vi "Prober_ProbeTouchdown.vi"(8 "error in (no error)":errorcluster, 11 "SemiProbe in":refnum<class "SemiProbe.lvclass">) -> (0 "error out":errorcluster, 1 "previous Z [µm]":i32, 2 "Z [µm]":i32, 3 "SemiProbe out":refnum<class "SemiProbe.lvclass">)   [LabVIEW 2018, in "SemiProbe.lvclass"]
uses:
  SemiProbe.lvclass
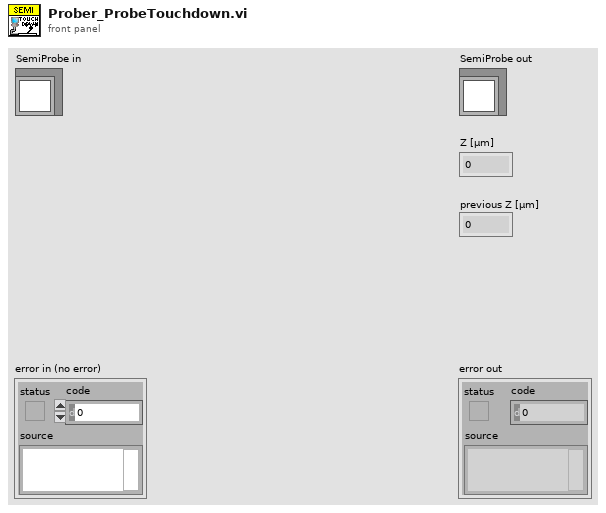
[diagram p1: front panel]
types:
  T1 = enum16{"Move To Load", "Move To Double Separation", "Move To Separation Distance", "Move To Contact", "Execute Contact Search", "Execute Arduino Contact Search"}
  T2 = cluster{"SP Load Less Than Thr?":bool, "SP Load Threshold (um)":dbl, "SP Current Location":cluster{"X (um)":ext, "Y (um)":ext, "Z (um)":ext, "T (degree)":ext}, "SP Chuck Speeds":cluster{"XY Speed (10-100%)":dbl, "Z Speed (10-100%)":dbl, "T Speed (10-100%)":dbl}, "Manual Step Parameters":cluster{"Step in X":bool, "X S-Speed [µm/step]":sgl, "Step in Y":bool, "Y S-Speed [µm/step]":sgl, "Step in Z":bool, "Z S-Speed [µm/step]":sgl, "Step in T":bool, "T S-Speed [mdegree/step]":sgl, "X Increase":bool, "Y Increase?":bool, "Z Increase?":bool, "T Increase?":bool}, "Z Stepper":cluster{"UP/DOWN":bool, "UP/DOWN Speed [µm/step]":i32, "SP Z Step":bool}, "Z Heights Set":bool, "SP Contact Search":cluster{"Contact Circuit":enum16{"12", "1", "2"}, "Speed [1000-10000]":sgl, "Start Height [µm]":sgl, "Search Band [µm]":sgl, "Overdrive [µm]":sgl}, "Separation Distance [µm]":u32, "Contact Height [µm]":u32, "Use Overdrive?":bool, "Touchdown method":enum16{"no feedback", "Arduino edgesense", "SP contact circuit"}, "Arduino Edgesense params":cluster{"touchdown height [µm]":i32, "search band [µm]":u32, "speed [µm/step]":u32, "overdrive [µm]":u32}}
  T3 = enum16{"no feedback", "Arduino edgesense", "SP contact circuit"}
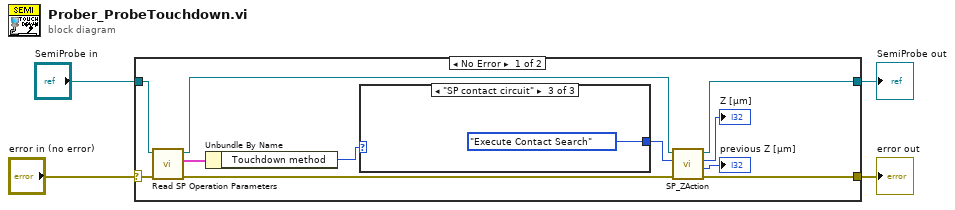
[diagram p0: block diagram]
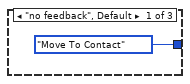
[diagram p2: hidden frame]
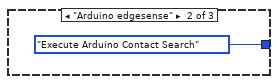
[diagram p3: hidden frame]
diagram:
  n1 = case shown="No Error" "error in (no error)" {
    selector: "error in (no error)" -> [w10 w19]
    tunnel: "SemiProbe in" -> [w9 w20]
    tunnel: [w12 w19] -> w2
    tunnel: [w11 w20] -> w1
    frame No Error {
      n2 = call-dynamic "Read SP Operation Parameters.vi"("error in (no error)"=w10, "SemiProbe in"=w9) -> ("error out"=w7:errorcluster, "SP Operation Parameters"=w6:T2, "SemiProbe out"=w8:refnum<class "SemiProbe.lvclass">)  [unwired: 7 in]
      n3 = Unbundle By Name(w6) -> ("Touchdown method"=w5:T3)
      n4 = case shown="\"SP contact circuit\"" w5 {
        tunnel: [T1."Move To Contact" ("Z Action") T1."Execute Arduino Contact Search" ("Z Action") T1."Execute Contact Search" ("Z Action")] -> w15
        frame "no feedback", Default {
        }
        frame "Arduino edgesense" {
        }
        frame "SP contact circuit" {
        }
      }
      n5 = call-dynamic "SP_ZAction.vi"("error in (no error)"=w7, "Z Action"=w15, "SemiProbe in"=w8) -> ("error out"=w12:errorcluster, "previous Z [µm]"=→"previous Z [µm]":i32, "Z [µm]"=→"Z [µm]":i32, "SemiProbe out"=w11:refnum<class "SemiProbe.lvclass">)  [unwired: 5 in]
    }
    frame Error {
    }
  }
  "error out" <- w2
  "SemiProbe out" <- w1
